vi "Configure Color Grade Analysis .vi"(6 "Color Grade Source (0: Channel 1)":i32(ring) items=["Channel 1", "Channel 2", "Channel 3", "Channel 4", "Math 1", "Math 2", "Math 3", "Math 4", "Reference Waveform 1", "Reference Waveform 2", "Reference Waveform 3", "Reference Waveform 4"], 7 "Color Grade Theme (0: Temperature)":i32(ring) items=["Temperature", "Intensity"], 8 "error in (no error)":errorcluster, 9 "Display Color Grade Key (T: Enable)":bool=TRUE, 10 "Enable Color Grade Analysis (T: Enable)":bool=TRUE, 11 "VISA resource name":refnum<visa-resource-name>) -> (0 "error out":errorcluster, 3 "VISA resource name out":refnum<visa-resource-name>)   [LabVIEW 2016, in "Agilent 2000 3000 X-Series.lvlib"]
doc: "Configures the color grade analysis feature.\n\n<b>Note:</b>\nThis VI is specific to the 6000-X Series oscilloscopes. These features are not available on other models."
uses:
  Agilent 2000 3000 X-Series.lvlib
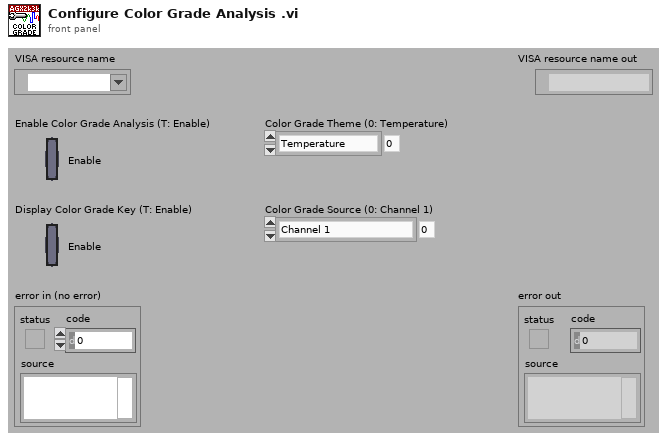
[diagram p1: front panel]
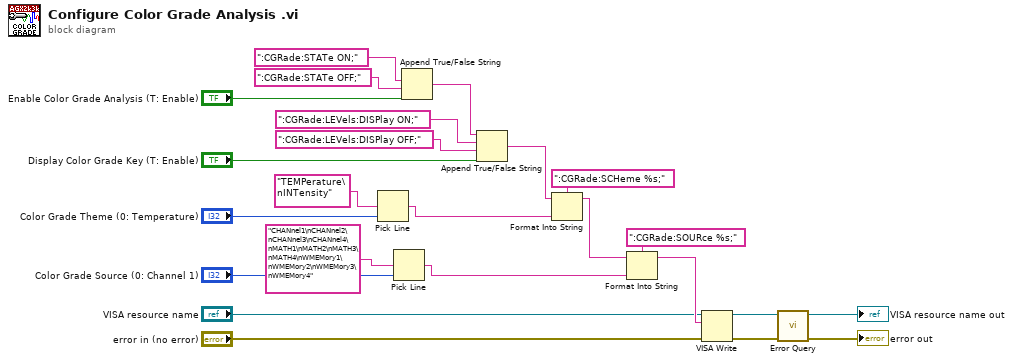
[diagram p0: block diagram]
diagram:
  n1 = Pick Line(multi-line string="TEMPerature\nINTensity", line index="Color Grade Theme (0: Temperature)") -> (output string=w8:string)  [unwired: 1 in]
  n2 = Pick Line(multi-line string="CHANnel1\nCHANnel2\nCHANnel3\nCHANnel4\nMATH1\nMATH2\nMATH3\nMATH4\nWMEMory1\nWMEMory2\nWMEMory3\nWMEMory4", line index="Color Grade Source (0: Channel 1)") -> (output string=w6:string)  [unwired: 1 in]
  n3 = Append True/False String(1:"Enable Color Grade Analysis (T: Enable)", 2:":CGRade:STATe OFF;", 3:":CGRade:STATe ON;") -> (0:w21:string)  [unwired: 1 in]
  n4 = Append True/False String(1:"Display Color Grade Key (T: Enable)", 2:":CGRade:LEVels:DISPlay OFF;", 3:":CGRade:LEVels:DISPlay ON;", 4:w21) -> (0:w17:string)
  n5 = Format Into String(format string=":CGRade:SCHeme %s;", initial string=w17, w8) -> (resulting string=w15:string)  [unwired: 1 in, 1 out]
  n6 = Format Into String(format string=":CGRade:SOURce %s;", initial string=w15, w6) -> (resulting string=w13:string)  [unwired: 1 in, 1 out]
  n7 = VISA Write(VISA resource name="VISA resource name", write buffer=w13, error in (no error)="error in (no error)") -> (VISA resource name out=w4:refnum<visa-resource-name>, error out=w3:errorcluster)  [unwired: 1 out]
  n8 = call "Error Query.vi"("error in (no error)"=w3, "VISA resource name"=w4) -> ("error out"=→"error out":errorcluster, "VISA resource name out"=→"VISA resource name out":refnum<visa-resource-name>)  [unwired: 6 in, 2 out]
